vi "CameraAngleCalib.vi"() -> ()   [LabVIEW 2019]
uses:
  <vilib>/userDefined/High Color/IMAQdx.ctl
  <vilib>/vision/NI_Vision_Development_Module.lvlib
panel:
  in  "error in (no error)":errorcluster
  in  "BackToInitail":string="G91\nG1 X-1.6703 Y-1.3974 F100"
  in  "ImageX2Y1":string="G91\nG1 X1.6703 Y0 F100"
  out "StichedImage2x1":T1(plugin-control)
  out "error out":errorcluster
  out "Image":T1[](array[plugin-control])
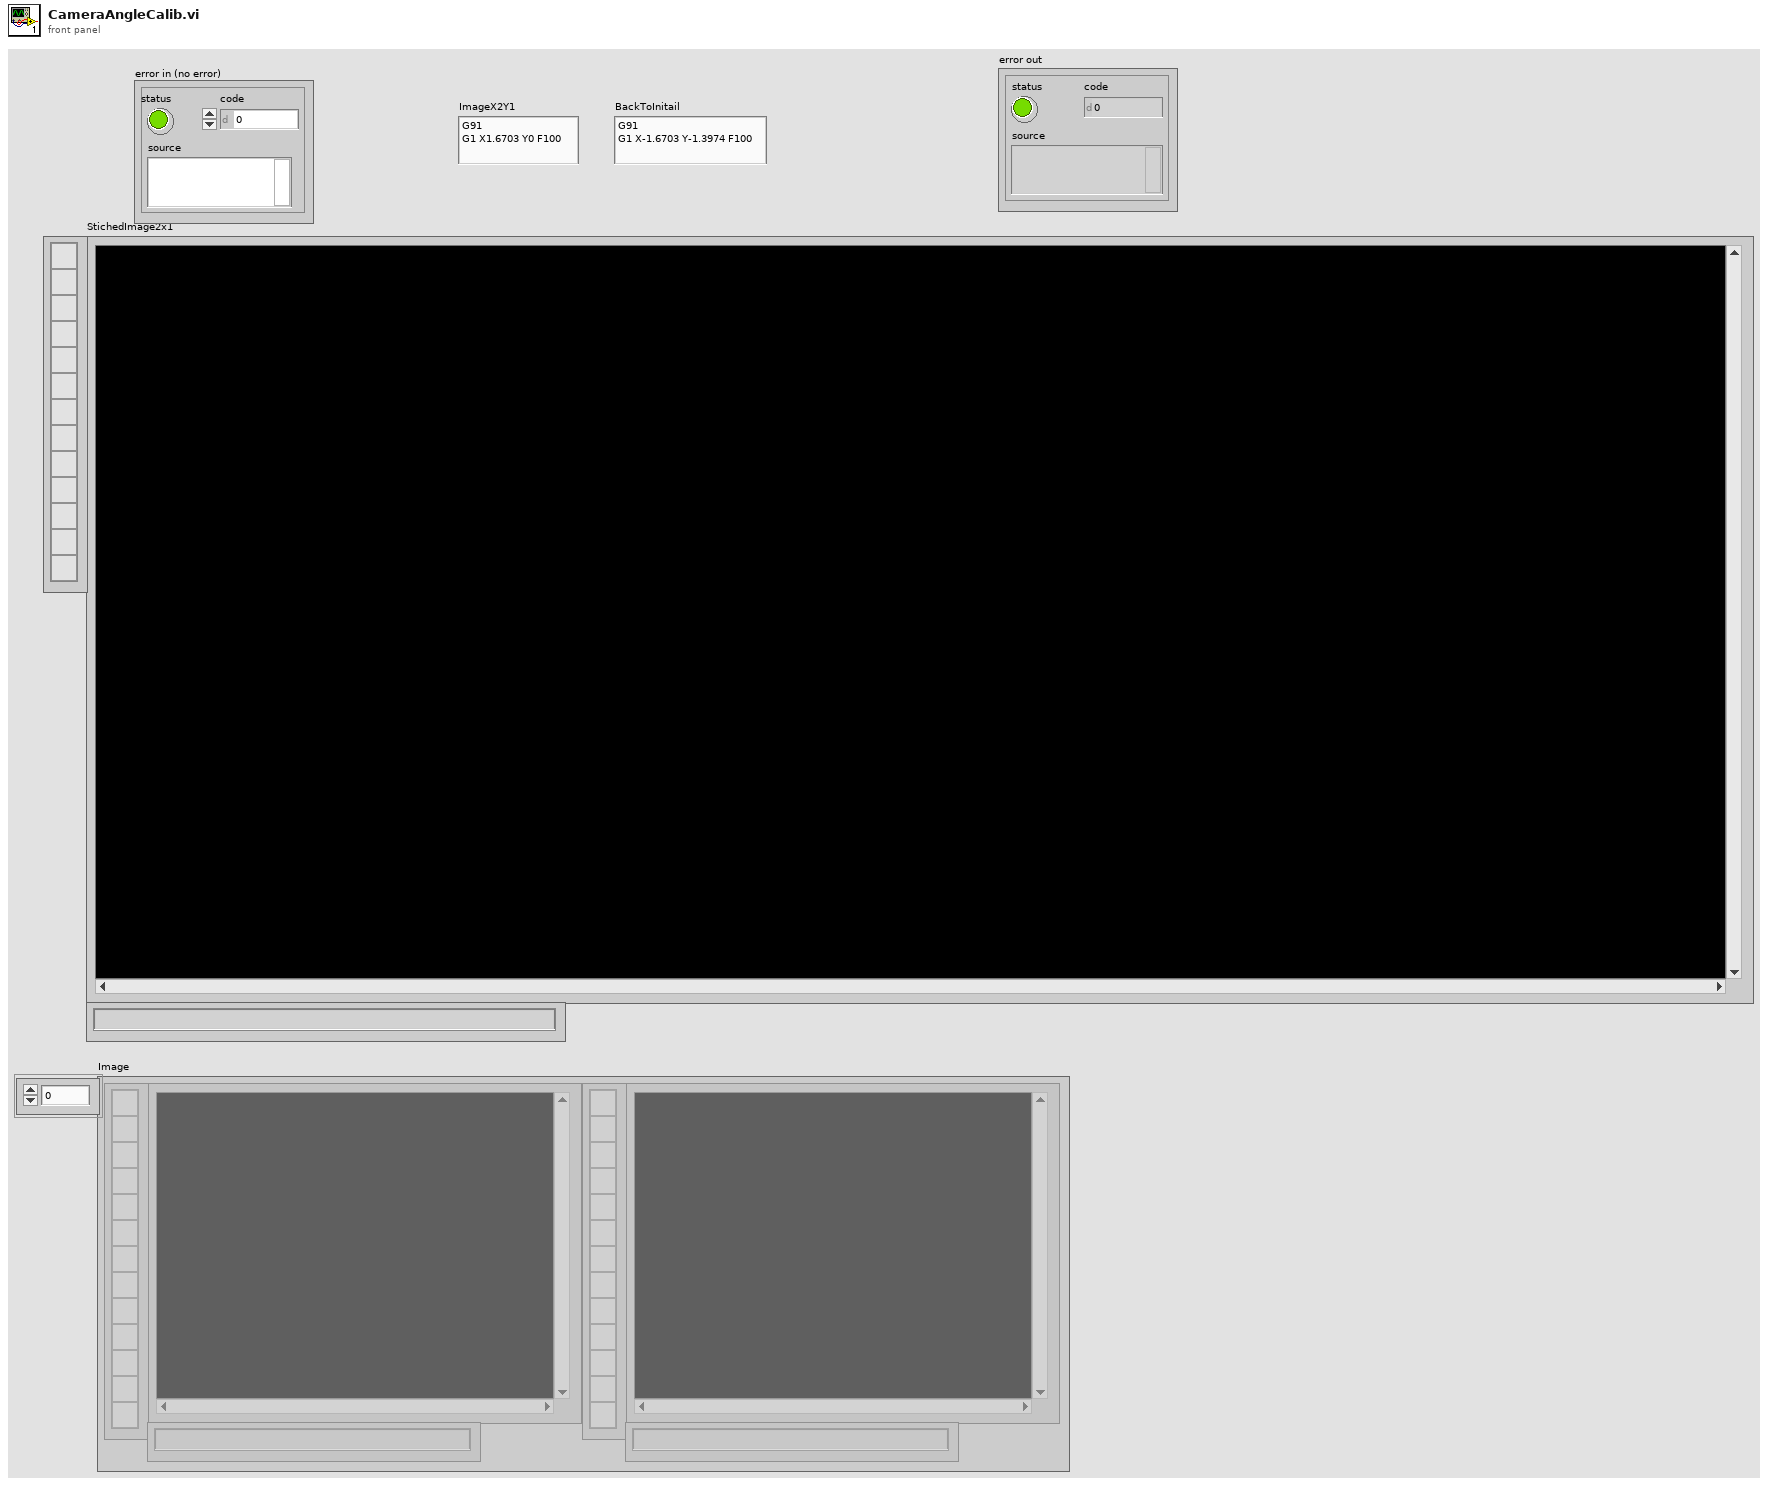
[diagram p1: front panel]
types:
  T1 = typedef "IMAQ Image.ctl" = refnum<image>
  T2 = typedef "IMAQdx.ctl" = refnum<k21>
  T3 = typedef "Image Type" = u32
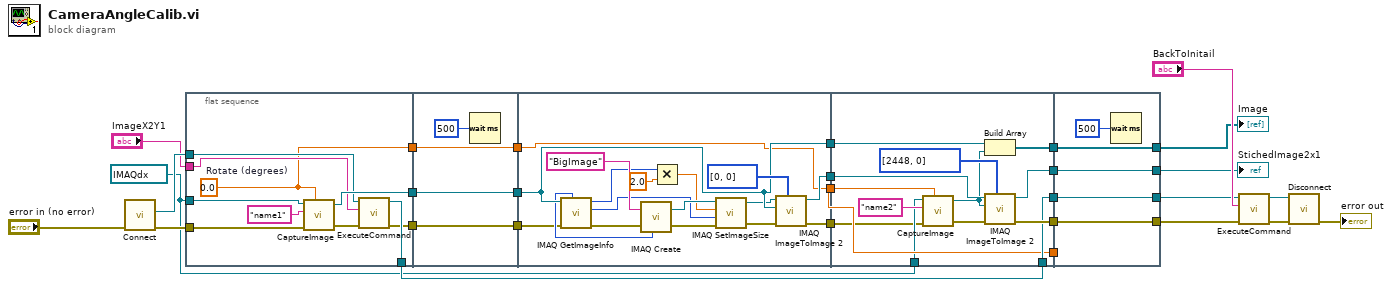
[diagram p0: block diagram]
diagram:
  w4 = T2 "cam1" ("Camera")
  n1 = call "Connect.vi"("error in (no error)"="error in (no error)") -> ("error out"=w26:errorcluster, "controller"=w23:refnum<k24>)  [unwired: 9 in]
  n2 = flat-sequence {
    tunnel: w4 -> [w38]
    tunnel: [w37] -> w25
    tunnel: w26 -> [w36]
    tunnel: w23 -> [w34]
    tunnel: "ImageX2Y1" -> [w33]
    tunnel: [w32] -> w16
    tunnel: [w31] -> w21
    tunnel: [w30] -> w17
    tunnel: w25 -> [w43]
    tunnel: [w43] -> w24
    tunnel: [w41] -> w22
    tunnel: w21 -> [w41]
    tunnel: [w40] -> w18
    tunnel: w17 -> [w40]
    tunnel: w24 -> [w56]
    tunnel: [w58] -> w29
    tunnel: [w56] -> w28
    tunnel: [w57] -> w27
    tunnel: w22 -> [w48]
    tunnel: [w47] -> w19
    tunnel: w18 -> [w47]
    tunnel: w16 -> [w70]
    tunnel: [w73] -> w14
    tunnel: [w72] -> w13
    tunnel: [w71] -> w12
    tunnel: [w70] -> w11
    tunnel: [w69] -> w10
    tunnel: w19 -> [w69]
    tunnel: w27 -> [w62]
    tunnel: w28 -> [w66]
    tunnel: w29 -> [w65]
    tunnel: w4 -> [w67]
    tunnel: w14 -> [w78]
    tunnel: w13 -> [w77]
    tunnel: w12 -> [w76]
    tunnel: w11 -> [w75]
    tunnel: w10 -> [_]
    tunnel: [w78] -> w2
    tunnel: [w77] -> w3
    tunnel: [w76] -> w6
    tunnel: [w75] -> w8
    frame #0 {
      w30 = sgl 0.0  # Rotate (degrees)
      n3 = call "CaptureImage.vi"("Camera"=w38, "Rotate (degrees)"=w30, "ImageName"="name1", "error in (no error)"=w36) -> ("Image"=w37:T1, "error out"=w35:errorcluster)  [unwired: 3 in]
      n4 = call "ExecuteCommand.vi"("error in (no error)"=w35, "Command Code"=w33, "controller in"=w34) -> ("error out"=w31:errorcluster, "controller out"=w32:refnum<k24>)  [unwired: 6 in, 1 out]
    }
    frame #1 {
      n5 = Wait (ms)(milliseconds to wait=u32 500) -> ()  [unwired: 1 out]
    }
    frame #2 {
      n6 = call "IMAQ GetImageInfo"("error in (no error)"=w48, "Image"=w56) -> ("error out"=w46:errorcluster, "Y Resolution"=w44:i32, "X Resolution"=w50:i32, "Image Type"=w55:T3)  [unwired: 2 in, 4 out]
      n7 = call "IMAQ Create"("Image Name"="BigImage", "Image Type"=w55, "error in (no error)"=w46) -> ("New Image"=w52:T1, "error out"=w54:errorcluster)  [unwired: 2 in]
      n8 = Multiply(x=w50, y=2.0) -> (x*y=w49:dbl)
      n9 = call "IMAQ SetImageSize"("error in (no error)"=w54, "Y Resolution"=w44, "X Resolution"=w49, "Image"=w52) -> ("error out"=w53:errorcluster, "Image Out"=w51:T1)  [unwired: 1 out]
      n10 = call "IMAQ ImageToImage 2"("Offset Left/Top"=i32[] [0, 0], "error in (no error)"=w53, "Image Src (Small)"=w56, "Image Src (Large)"=w51) -> ("error out"=w58:errorcluster, "Image Dst Out"=w57:T1)  [unwired: 2 in, 4 out]
    }
    frame #3 {
      n11 = call "CaptureImage.vi"("Camera"=w67, "Rotate (degrees)"=w69, "ImageName"="name2", "error in (no error)"=w65) -> ("Image"=w61:T1, "error out"=w63:errorcluster)  [unwired: 3 in]
      n12 = Build Array(w66, w61) -> (w73:T1[])
      n13 = call "IMAQ ImageToImage 2"("Offset Left/Top"=i32[] [2448, 0], "error in (no error)"=w63, "Image Src (Small)"=w61, "Image Src (Large)"=w62) -> ("error out"=w71:errorcluster, "Image Dst Out"=w72:T1)  [unwired: 2 in, 4 out]
    }
    frame #4 {
      n14 = Wait (ms)(milliseconds to wait=u32 500) -> ()  [unwired: 1 out]
    }
  }
  n15 = call "ExecuteCommand.vi"("error in (no error)"=w6, "Command Code"="BackToInitail", "controller in"=w8) -> ("error out"=w5:errorcluster, "controller out"=w7:refnum<k24>)  [unwired: 6 in, 1 out]
  n16 = call "Disconnect.vi"("error in (no error)"=w5, "controller"=w7) -> ("error out"=→"error out":errorcluster)  [unwired: 9 in]
  "Image" <- w2
  "StichedImage2x1" <- w3
